vi "Tester.vi"() -> ()   [LabVIEW 2019, in "Logger.lvclass"]
uses:
  Logger.lvclass
  IAction/IAction.lvclass
  IConfig/IConfig.lvclass
  IReference/IReference.lvclass
  IResult/IResult.lvclass
panel:
  out "Timeout?":bool
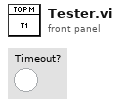
[diagram p1: front panel]
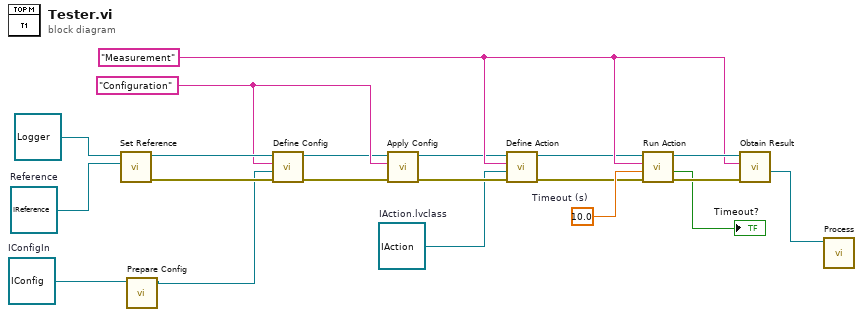
[diagram p0: block diagram]
diagram:
  w2 = refnum<class "IReference.lvclass"> refnum  # Reference
  w3 = refnum<class "IConfig.lvclass"> refnum  # IConfigIn
  w4 = refnum<class "IAction.lvclass"> refnum  # IAction.lvclass
  w15 = 10.0  # Timeout (s)
  w14 = "Measurement" ("Name")
  w19 = "Configuration" ("Name")
  n1 = call "Set Reference.vi"("Reference"=w2, "Logger In"=refnum<class "Logger.lvclass"> refnum ("Logger.lvclass")) -> ("Error Out"=w18:errorcluster, "Logger Out"=w20:refnum<class "Logger.lvclass">)  [unwired: 8 in]
  n2 = call-dynamic "Prepare Config.vi"("IConfigIn"=w3) -> ("IConfigOut"=w5:refnum<class "IConfig.lvclass">)  [unwired: 9 in, 1 out]
  n3 = call "Define Config.vi"("Error In"=w18, "Config"=w5, "Name"=w19, "Logger In"=w20) -> ("Error Out"=w12:errorcluster, "Logger Out"=w13:refnum<class "Logger.lvclass">)  [unwired: 6 in]
  n4 = call "Apply Config.vi"("ErrorIn"=w12, "Name"=w19, "TopModuleIn"=w13) -> ("ErrorOut"=w10:errorcluster, "TopModuleOut"=w11:refnum<class "Logger.lvclass">)  [unwired: 7 in]
  n5 = call "Define Action.vi"("Error In"=w10, "Measurement"=w4, "Name"=w14, "Logger In"=w11) -> ("Error Out"=w8:errorcluster, "Logger Out"=w9:refnum<class "Logger.lvclass">)  [unwired: 6 in]
  n6 = call "Run Action.vi"("Error In"=w8, "Timeout (s)"=w15, "Action"=w14, "Logger In"=w9) -> ("Error Out"=w16:errorcluster, "Timeout?"=→"Timeout?":bool, "Logger Out"=w17:refnum<class "Logger.lvclass">)  [unwired: 5 in]
  n7 = call "Obtain Result.vi"("Error In"=w16, "Name"=w14, "Logger In"=w17) -> ("Result Out"=w7:refnum<class "IResult.lvclass">)  [unwired: 5 in, 3 out]
  n8 = call-dynamic "Process.vi"("IResultIn"=w7) -> ()  [unwired: 9 in, 2 out]
